vi "Field Handle Operator Notes.vi"(8 "error in (no error)":errorcluster, 9 "on Fail? (f = on Repeat)":bool, 10 "Sequence ID (\"\")":string, 11 "Connection Refnum":T4) -> (0 "error out":errorcluster, 2 "Operator Note on Repeat Field":T1={"ixField"=0, "iSequenceOrder"=0, "sxFieldId"="", "sxSequenceId"="", "sDisplayName"="", "sValue"="", "sUnits"="", "nDataType"=enum."timestamp", "nNextItem"=enum."Reset", "fSystem"=FALSE, "fSystemValue"=FALSE, "fRequired"=FALSE, "fSetAtTest"=FALSE, "fTestField"=FALSE, "fDeleted"=FALSE, "fIndexed"=FALSE, "fFreeList"=FALSE}, 3 "Connection Refnum":T4)   [LabVIEW 2011]
uses:
  Field System Fields.ctl
  Field Record.ctl
  Field NextItem.ctl
  Field DataTypes.ctl
  SI.LIB/ODBC/SQL Controls/Connection Refnum.ctl
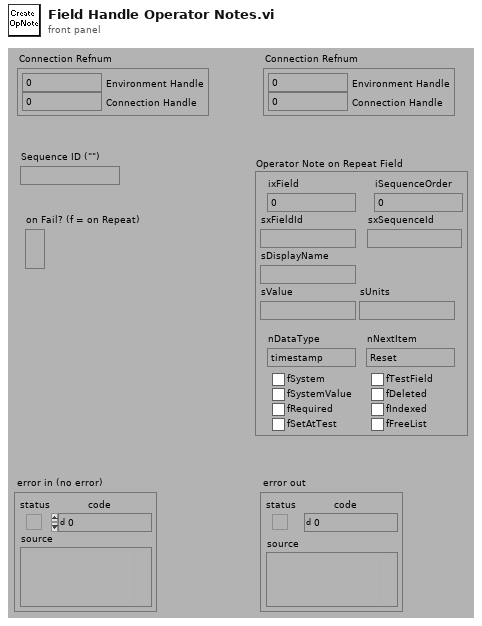
[diagram p1: front panel]
types:
  T1 = typedef "Field Record.ctl" = cluster{"ixField":i32, "iSequenceOrder":i32, "sxFieldId":string, "sxSequenceId":string, "sDisplayName":string, "sValue":string, "sUnits":string, "nDataType":T2, "nNextItem":T3, "fSystem":bool, "fSystemValue":bool, "fRequired":bool, "fSetAtTest":bool, "fTestField":bool, "fDeleted":bool, "fIndexed":bool, "fFreeList":bool}
  T2 = typedef "Field DataTypes.ctl" = enum32{"text", "numeric", "list", "timestamp", "boolean"}
  T3 = typedef "Field NextItem.ctl" = enum32{"Reset", "Retain", "Auto-Increment"}
  T4 = typedef "Connection Refnum.ctl" = cluster{"Environment Handle":i32, "Connection Handle":i32}
  T5 = typedef "Field System Fields.ctl" = enum32{"Company", "End_Timestamp", "Model_Number", "Operator", "Serial_Number", "Start_Timestamp", "Step_Number", "Step_Tag", "Test_Run", "Test_Sequence", "Test_Station", "Test_Station_Name", "Test_Status", "Test_Type", "Test_Version", "Spartan_Version_Created", "Spartan_Version_Current"}
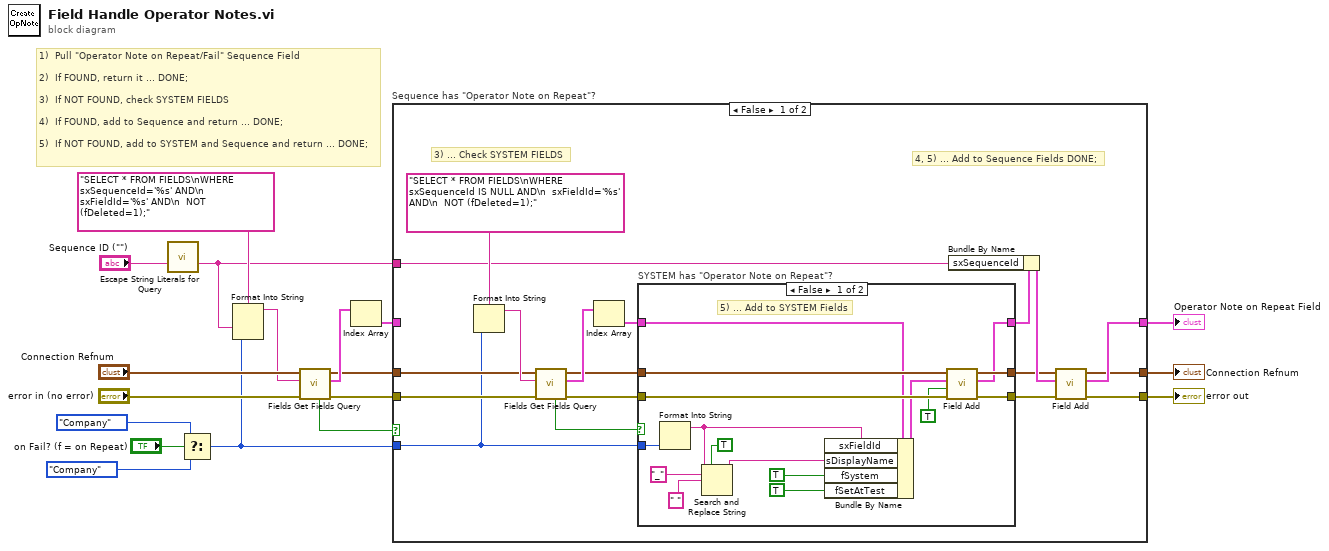
[diagram p0: block diagram]
diagram:
  # "1)  Pull \"Operator Note on Repeat/Fail\" Sequence Field\n\n2)  If FOUND, return it ... DONE;\n\n3)  If NOT FOUND, check SYSTEM FIELDS\n\n4)  If FOUND, add to Sequence and return ... DONE;\n\n5)  If NOT FOUND, add to SYSTEM and Sequence and return ... DONE;"
  n1 = call "Escape String Literals for Query.vi"("String"="Sequence ID (\"\")") -> ("escaped String"=w5:string)  [unwired: 1 in, 13 out]
  n2 = Select(t=Field_System_Fields."Company" ("System Fields"), s="on Fail? (f = on Repeat)", f=Field_System_Fields."Company" ("System Fields")) -> (s? t:f=w4:T5)
  n3 = Format Into String(format string="SELECT * FROM FIELDS\nWHERE sxSequenceId='%s' AND\n  sxFieldId='%s' AND\n  NOT (fDeleted=1);", w5, w4) -> (resulting string=w14:string)  [unwired: 2 in, 1 out]
  n4 = call "Fields Get Fields Query.vi"("error in (no error)"="error in (no error)", "Query"=w14, "Connection Refnum"="Connection Refnum") -> ("error out"=w9:errorcluster, "Fields"=w12:T1[], "Connection Refnum"=w10:T4, "Data Present?"=w13:bool)  [unwired: 5 out]
  n5 = Index Array(array=w12) -> (element=w11:T1)  [unwired: 1 in]
  n6 = case "Sequence has \"Operator Note on Repeat\"?" shown="False" w13 {
    tunnel: w11 -> [_ w58]
    tunnel: w10 -> [w34 w57]
    tunnel: w9 -> [w33 w56]
    tunnel: [w31 w58] -> w8
    tunnel: [w28 w57] -> w7
    tunnel: [w27 w56] -> w6
    tunnel: w4 -> [w19 _]
    tunnel: w5 -> [w30 _]
    frame False {
      # "4, 5) ... Add to Sequence Fields DONE;"
      # "3) ... Check SYSTEM FIELDS"
      n7 = Format Into String(format string="SELECT * FROM FIELDS\nWHERE sxSequenceId IS NULL AND\n  sxFieldId='%s' AND\n  NOT (fDeleted=1);", w19) -> (resulting string=w36:string)  [unwired: 2 in, 1 out]
      n8 = call "Fields Get Fields Query.vi"("error in (no error)"=w33, "Query"=w36, "Connection Refnum"=w34) -> ("error out"=w22:errorcluster, "Fields"=w32:T1[], "Connection Refnum"=w23:T4, "Data Present?"=w26:bool)  [unwired: 5 out]
      n9 = Index Array(array=w32) -> (element=w25:T1)  [unwired: 1 in]
      n10 = case "SYSTEM has \"Operator Note on Repeat\"?" shown="False" w26 {
        tunnel: w25 -> [w47 w55]
        tunnel: [w48 w55] -> w24
        tunnel: w23 -> [w52 w54]
        tunnel: w22 -> [w51 w53]
        tunnel: [w50 w54] -> w21
        tunnel: [w49 w53] -> w20
        tunnel: w19 -> [w42 _]
        frame False {
          # "5) ... Add to SYSTEM Fields"
          n11 = Format Into String(w42) -> (resulting string=w41:string)  [unwired: 3 in, 1 out]
          n12 = Search and Replace String(replace all?=TRUE, input string=w41, search string="_", replace string=" " ("search string")) -> (result string=w40:string)  [unwired: 1 in, 6 out]
          n13 = Bundle By Name(cluster=w47, "sxFieldId"=w41, "sDisplayName"=w40, "fSystem"=TRUE, "fSetAtTest"=TRUE) -> (w44:T1)
          n14 = call "Field Add.vi"("error in (no error)"=w51, "Force Unique? (f)"=TRUE, "Field Record"=w44, "Connection Refnum"=w52) -> ("error out"=w49:errorcluster, "New Field"=w48:T1, "Connection Refnum"=w50:T4)  [unwired: 5 out]
        }
        frame True {
        }
      }
      n15 = Bundle By Name(cluster=w24, "sxSequenceId"=w30) -> (w29:T1)
      n16 = call "Field Add.vi"("error in (no error)"=w20, "Field Record"=w29, "Connection Refnum"=w21) -> ("error out"=w27:errorcluster, "New Field"=w31:T1, "Connection Refnum"=w28:T4)  [unwired: 1 in, 5 out]
    }
    frame True {
      # "2) ... DONE"
    }
  }
  "error out" <- w6
  "Connection Refnum" <- w7
  "Operator Note on Repeat Field" <- w8
